vi "test Sort Array of Clusters.vi"(8 "error in (no error)":errorcluster, 11 "TestCase in":refnum<class "UI Common Unit Tests.lvclass">) -> (0 "error out":errorcluster, 3 "TestCase out":refnum<class "UI Common Unit Tests.lvclass">)   [LabVIEW 2020, in "UI Common Unit Tests.lvclass"]
uses:
  UI Common Unit Tests.lvclass
  Array Row.ctl
  63dc8703-c824-4b80-a085-58f57073aca5.vi
  d8dc5a30-59fd-40f1-b092-92b0634dc405.vi
  c62d43f3-ccf2-448e-89d3-d67a32af4b30.vi
  0d07b81e-88f3-4258-8836-385d3b76f707.vi
  63dc8703-c824-4b80-a085-58f57073aca5.vi/c6e47537-c08d-48c3-af9a-650f4b7d2927.vi
  63dc8703-c824-4b80-a085-58f57073aca5.vi/05f20fbf-b3a3-4cd2-83ab-c2f9dc8feb5b.vi
  d8dc5a30-59fd-40f1-b092-92b0634dc405.vi/6bbd4f04-926b-4bf8-b987-18fced4156cc.vi
  d8dc5a30-59fd-40f1-b092-92b0634dc405.vi/feb5878f-735b-445c-a802-e95ef67c9eb4.vi
  c62d43f3-ccf2-448e-89d3-d67a32af4b30.vi/f5199f28-757e-4dca-8f31-ba679ec209f5.vi
  c62d43f3-ccf2-448e-89d3-d67a32af4b30.vi/e57e02eb-0b74-48ac-a850-073f97e4d6e8.vi
  0d07b81e-88f3-4258-8836-385d3b76f707.vi/1563cfa7-633d-4947-b146-ce80bb5c8354.vi
  0d07b81e-88f3-4258-8836-385d3b76f707.vi/4a272fd0-111f-404a-ba1b-72b108e1c79f.vi
  Natural String Merge Sort.vi
  <vilib>/addons/_JKI Toolkits/VI Tester/TestCase.llb/TestCase.lvclass
  C:/Program Files (x86)/National Instruments/LabVIEW 2020/vi.lib/addons/_JKI Toolkits/VI Tester/TestCase.llb/TestCase.lvclass
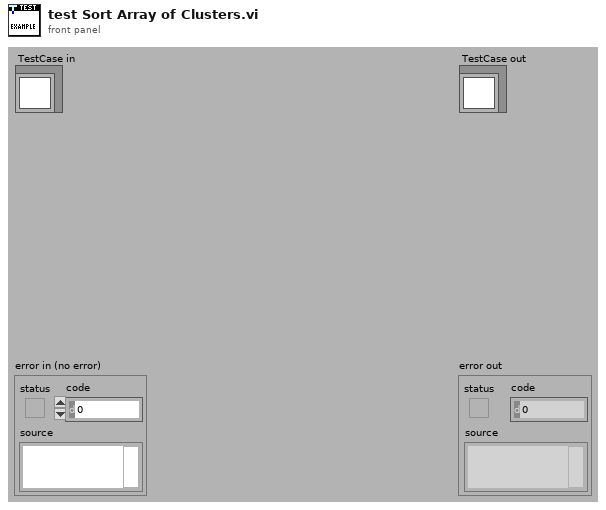
[diagram p1: front panel]
types:
  T1 = typedef "UI Common Unit Tests.lvclass/Array Row.ctl" = cluster{"String":string, "Numeric":dbl}
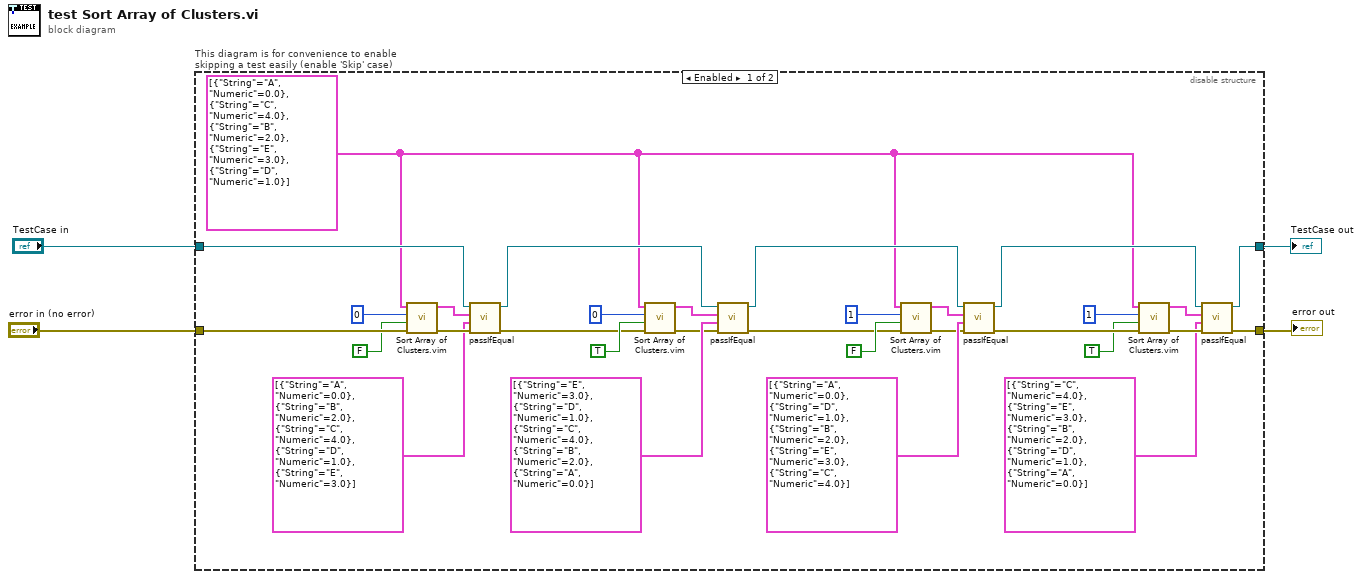
[diagram p0: block diagram]
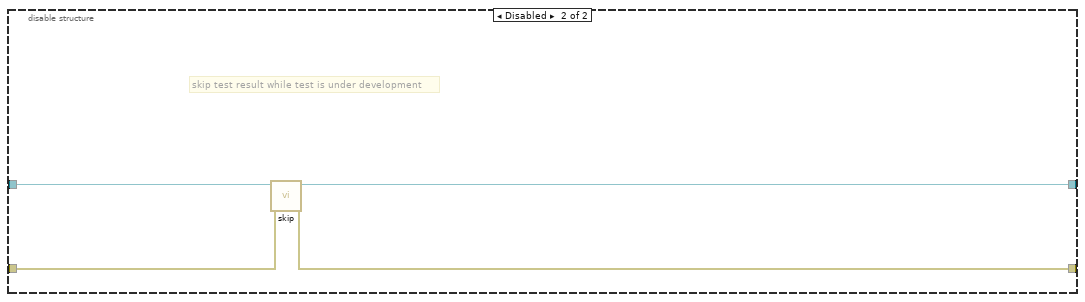
[diagram p2: hidden frame]
diagram:
  n1 = disable-structure "This diagram is for convenience to enable skipping a test easily (enable 'Skip' case)" shown="Enabled" {
    disable-tunnel: "TestCase in" -> [w31 w39]
    disable-tunnel: [w10 w37] -> w1
    disable-tunnel: [w6 w38] -> w3
    disable-tunnel: "error in (no error)" -> [w35 w36]
    frame Enabled {
      w5 = T1[] [{"String"="A", "Numeric"=0.0}, {"String"="C", "Numeric"=4.0}, {"String"="B", "Numeric"=2.0}, {"String"="E", "Numeric"=3.0}, {"String"="D", "Numeric"=1.0}] ("Value")
      n2 = call "Sort Array of Clusters.vim"("error in (no error)"=w35, "Descending"=FALSE, "index"=u32 0, "Array"=w5) -> ("error out"=w32:errorcluster, "Sorted Array"=w30:T1[])  [unwired: 6 in]
      n3 = call-dynamic "passIfEqual.vi"("error in (no error)"=w32, "y"=T1[] [{"String"="A", "Numeric"=0.0}, {"String"="B", "Numeric"=2.0}, {"String"="C", "Numeric"=4.0}, {"String"="D", "Numeric"=1.0}, {"String"="E", "Numeric"=3.0}] ("Value"), "x"=w30, "TestCase in"=w31) -> ("error out"=w23:errorcluster, "TestCase out"=w22:refnum<class "UI Common Unit Tests.lvclass">)  [unwired: 6 in]
      n4 = call "Sort Array of Clusters.vim"("error in (no error)"=w23, "Descending"=TRUE, "index"=u32 0, "Array"=w5) -> ("error out"=w26:errorcluster, "Sorted Array"=w27:T1[])  [unwired: 6 in]
      n5 = call-dynamic "passIfEqual.vi"("error in (no error)"=w26, "y"=T1[] [{"String"="E", "Numeric"=3.0}, {"String"="D", "Numeric"=1.0}, {"String"="C", "Numeric"=4.0}, {"String"="B", "Numeric"=2.0}, {"String"="A", "Numeric"=0.0}] ("Value"), "x"=w27, "TestCase in"=w22) -> ("error out"=w7:errorcluster, "TestCase out"=w8:refnum<class "UI Common Unit Tests.lvclass">)  [unwired: 6 in]
      n6 = call "Sort Array of Clusters.vim"("error in (no error)"=w7, "Descending"=FALSE, "index"=u32 1, "Array"=w5) -> ("error out"=w13:errorcluster, "Sorted Array"=w14:T1[])  [unwired: 6 in]
      n7 = call-dynamic "passIfEqual.vi"("error in (no error)"=w13, "y"=T1[] [{"String"="A", "Numeric"=0.0}, {"String"="D", "Numeric"=1.0}, {"String"="B", "Numeric"=2.0}, {"String"="E", "Numeric"=3.0}, {"String"="C", "Numeric"=4.0}] ("Value"), "x"=w14, "TestCase in"=w8) -> ("error out"=w21:errorcluster, "TestCase out"=w9:refnum<class "UI Common Unit Tests.lvclass">)  [unwired: 6 in]
      n8 = call "Sort Array of Clusters.vim"("error in (no error)"=w21, "Descending"=TRUE, "index"=u32 1, "Array"=w5) -> ("error out"=w18:errorcluster, "Sorted Array"=w17:T1[])  [unwired: 6 in]
      n9 = call-dynamic "passIfEqual.vi"("error in (no error)"=w18, "y"=T1[] [{"String"="C", "Numeric"=4.0}, {"String"="E", "Numeric"=3.0}, {"String"="B", "Numeric"=2.0}, {"String"="D", "Numeric"=1.0}, {"String"="A", "Numeric"=0.0}] ("Value"), "x"=w17, "TestCase in"=w9) -> ("error out"=w6:errorcluster, "TestCase out"=w10:refnum<class "UI Common Unit Tests.lvclass">)  [unwired: 6 in]
    }
    frame Disabled {
      # "skip test result while test is under development"
      n10 = call <vilib>:"skip.vi"("error in (no error)"=w36, "TestCase in"=w39) -> ("error out"=w38:errorcluster, "TestCase out"=w37:refnum<class "UI Common Unit Tests.lvclass">)  [unwired: 8 in]
    }
  }
  "error out" <- w3
  "TestCase out" <- w1
